vi "start.vi"(8 "error in (no error)":errorcluster, 10 "model":refnum<class "Model.lvclass">, 11 "StandbyState in":refnum<class "StandbyState.lvclass">) -> (0 "error out":errorcluster, 2 "model 2":refnum<class "Model.lvclass">, 3 "StandbyState out":refnum<class "StandbyState.lvclass">)   [LabVIEW 2013, in "StandbyState.lvclass"]
uses:
  StandbyState.lvclass
  Model/Model/Model.lvclass
  Typedefs/StateSelector.ctl
  Typedefs/M2AADTTypedefs.lvlib
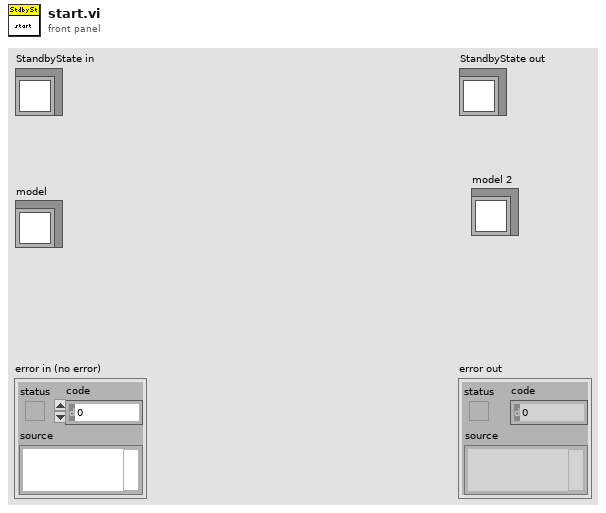
[diagram p1: front panel]
types:
  T1 = typedef "M2AADTTypedefs.lvlib/StateSelector.ctl" = enum16{"EndingCycleState", "FaultState", "InteractiveMotionState", "MovingToNewForceState", "OffState", "PausingState", "StandbyState", "StoppedState"}
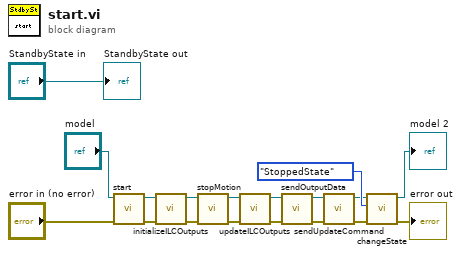
[diagram p0: block diagram]
diagram:
  n1 = call "start.vi"("error in (no error)"="error in (no error)", "Model in"="model") -> ("error out"=w10:errorcluster, "Model out"=w12:refnum<class "Model.lvclass">)  [unwired: 8 in]
  n2 = call "initializeILCOutputs.vi"("error in (no error)"=w10, "Model in"=w12) -> ("error out"=w9:errorcluster, "Model out"=w11:refnum<class "Model.lvclass">)  [unwired: 8 in]
  n3 = call "stopMotion.vi"("error in (no error)"=w9, "Model in"=w11) -> ("error out"=w6:errorcluster, "Model out"=w8:refnum<class "Model.lvclass">)  [unwired: 8 in]
  n4 = call "updateILCOutputs.vi"("error in (no error)"=w6, "Model in"=w8) -> ("error out"=w5:errorcluster, "Model out"=w7:refnum<class "Model.lvclass">)  [unwired: 8 in]
  n5 = call "sendOutputData.vi"("error in (no error)"=w5, "Model in"=w7) -> ("error out"=w1:errorcluster, "Model out"=w2:refnum<class "Model.lvclass">)  [unwired: 8 in]
  n6 = call "sendUpdateCommand.vi"("error in (no error)"=w1, "Model in"=w2) -> ("error out"=w3:errorcluster, "Model out"=w4:refnum<class "Model.lvclass">)  [unwired: 8 in]
  n7 = call "changeState.vi"("error in (no error)"=w3, "State:"=StateSelector."StoppedState", "Model in"=w4) -> ("error out"=→"error out":errorcluster, "Model out"=→"model 2":refnum<class "Model.lvclass">)  [unwired: 7 in]
  "StandbyState out" <- "StandbyState in"
